vi "Server_API_Call.vi"(6 "Server":path, 7 "Direction":enum16{"ASK", "TELL"}(ring), 8 "error in (no error)":errorcluster, 9 "Payload":string, 11 "cmd":string) -> (0 "error out":errorcluster, 1 "Running?":bool, 2 "Send to Server":string, 3 "Read from Server":string)   [LabVIEW 2020]
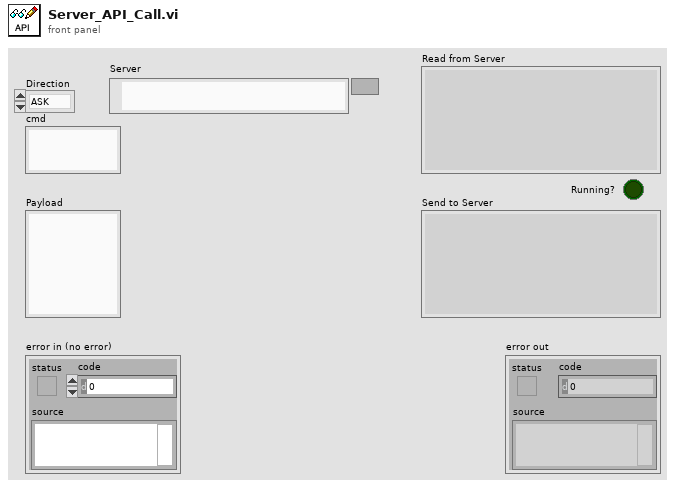
[diagram p1: front panel]
types:
  T1 = enum32{"Bad", "Idle", "Run top level", "Running"}
  T2 = enum32{"Invalid", "Standard", "Closed", "Hidden", "Minimized", "Maximized"}
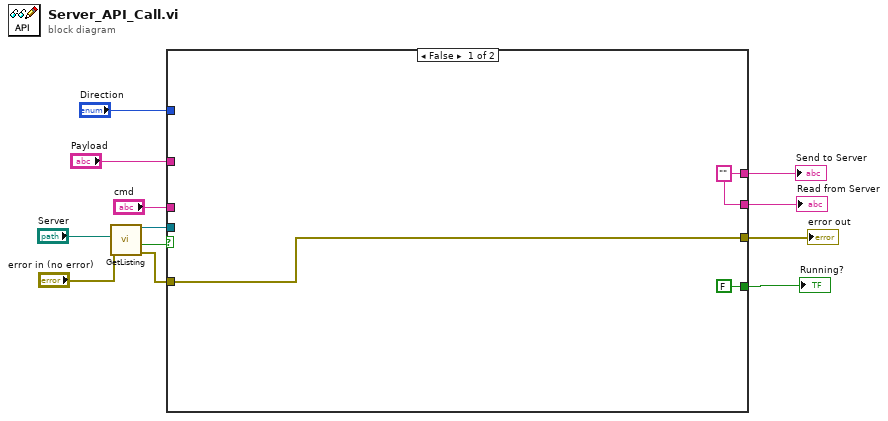
[diagram p0: block diagram]
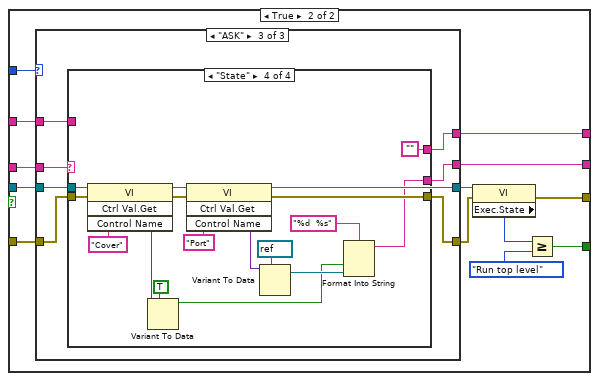
[diagram p2: hidden frame]
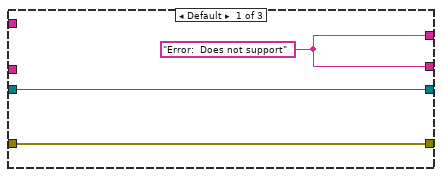
[diagram p3: hidden frame]
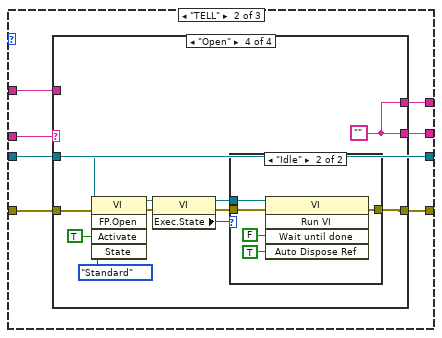
[diagram p4: hidden frame]
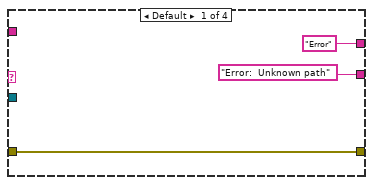
[diagram p5: hidden frame]
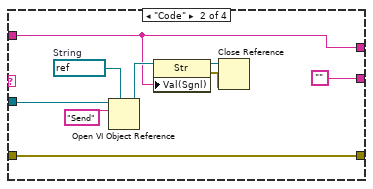
[diagram p6: hidden frame]
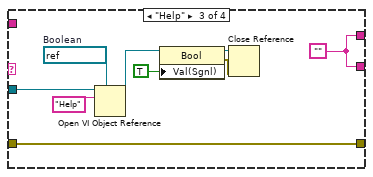
[diagram p7: hidden frame]
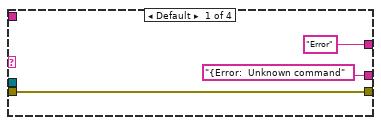
[diagram p9: hidden frame]
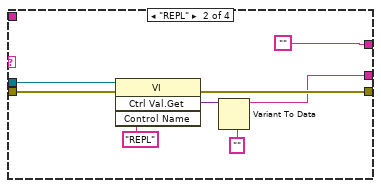
[diagram p10: hidden frame]
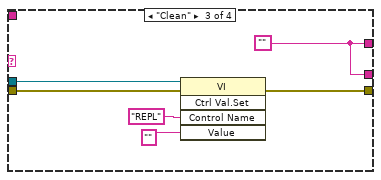
[diagram p11: hidden frame]
diagram:
  n1 = call "GetListing.vi"("error in (no error)"="error in (no error)", "Server"="Server") -> ("error out"=w4:errorcluster, "Found"=w1:bool, "VI out"=w9:refnum<vi>)  [unwired: 7 in]
  n2 = case shown="False" w1 {
    tunnel: [w15 w28] -> w12
    tunnel: [w15 w27] -> w11
    tunnel: w9 -> [_ w26]
    tunnel: "Direction" -> [_ w25]
    tunnel: "Payload" -> [_ w24]
    tunnel: "cmd" -> [_ w23]
    tunnel: w4 -> [w14 w22]
    tunnel: [FALSE w17] -> w3
    tunnel: [w14 w16] -> w2
    frame False {
      w15 = "" ("input 2")
    }
    frame True {
      n3 = case shown="\"ASK\"" w25 {
        tunnel: [w31 w38 w83] -> w28
        tunnel: w24 -> [_ w37 w82]
        tunnel: [w31 w36 w81] -> w27
        tunnel: w26 -> [w29 w32 w77]
        tunnel: w22 -> [w30 w35 w80]
        tunnel: [w30 w34 w79] -> w20
        tunnel: w23 -> [_ w33 w78]
        tunnel: [w29 w32 w77] -> w21
        frame Default {
          w31 = "Error:  Does not support" ("input 2")
        }
        frame "TELL" {
          n4 = case shown="\"Open\"" w33 {
            tunnel: ["Error:  Unknown path" ("input 2") "" w51 w68] -> w38
            tunnel: w37 -> [_ w44 _ _]
            tunnel: ["Error" ("input 2") w44 w51 w68] -> w36
            tunnel: w35 -> [w39 w49 w59 w66]
            tunnel: [w39 w49 w59 w60] -> w34
            tunnel: w32 -> [_ w46 w56 w67]
            frame Default {
            }
            frame "Code" {
              w48 = refnum<vi> refnum  # String
              n5 = Open VI Object Reference(7:w48, 10:"Send" ("name/order"), 11:w46) -> (3:w45:refnum<vi>)  [unwired: 1 in, 1 out]
              n6 = property class="Str"(reference=w45, "Val(Sgnl)"=w44) -> (reference out=w42:refnum<vi>, error out=w43:errorcluster)  [unwired: 1 in]
              n7 = Close Reference(reference=w42, error in (no error)=w43) -> ()  [unwired: 1 out]
            }
            frame "Help" {
              w58 = refnum<vi> refnum  # Boolean
              w51 = ""
              n8 = Open VI Object Reference(7:w58, 10:"Help" ("name/order"), 11:w56) -> (3:w55:refnum<vi>)  [unwired: 1 in, 1 out]
              n9 = property class="Bool"(reference=w55, "Val(Sgnl)"=TRUE) -> (reference out=w53:refnum<vi>, error out=w54:errorcluster)  [unwired: 1 in]
              n10 = Close Reference(reference=w53, error in (no error)=w54) -> ()  [unwired: 1 out]
            }
            frame "Open" {
              w68 = ""
              n11 = invoke class="VI" method="FP.Open"(reference=w67, error in=w66, "Activate"=TRUE ("Activate?"), "State"=T2."Standard" ("Front Panel Window:State")) -> (reference out=w65:refnum<vi>, error out=w64:errorcluster)  [unwired: 1 in, 3 out]
              n12 = property class="VI"(reference=w65, error in=w64) -> (reference out=w62:refnum<vi>, error out=w61:errorcluster, "Exec.State"=w63:T1)
              n13 = case shown="\"Idle\"" w63 {
                tunnel: w62 -> [_ w76]
                tunnel: w61 -> [w71 w75]
                tunnel: [w71 w74] -> w60
                frame Default {
                }
                frame "Idle" {
                  n14 = invoke class="VI" method="Run VI"(reference=w76, error in=w75, "Wait until done"=FALSE ("Activate?"), "Auto Dispose Ref"=TRUE ("Activate?")) -> (error out=w74:errorcluster)  [unwired: 1 in, 4 out]
                }
              }
            }
          }
        }
        frame "ASK" {
          n15 = case shown="\"State\"" w78 {
            tunnel: ["{Error:  Unknown command" ("input 2") w87 w100 w101] -> w83
            tunnel: w82 -> [_ _ _ _]
            tunnel: ["Error" ("input 2") "" w100 ""] -> w81
            tunnel: w77 -> [_ w89 w97 w109]
            tunnel: w80 -> [w84 w90 w96 w108]
            tunnel: [w84 w88 w95 w105] -> w79
            frame Default {
            }
            frame "REPL" {
              n16 = invoke class="VI" method="Ctrl Val.Get"(reference=w89, error in=w90, "Control Name"="REPL") -> (error out=w88:errorcluster, "Get Control Value Variant"=w92:variant)  [unwired: 1 in, 2 out]
              n17 = Variant To Data(type="" ("Control Name"), Variant=w92) -> (data=w87:string)  [unwired: 1 in, 1 out]
            }
            frame "Clean" {
              w100 = ""
              n18 = invoke class="VI" method="Ctrl Val.Set"(reference=w97, error in=w96, "Control Name"="REPL", "Value"="" ("Control Name")) -> (error out=w95:errorcluster)  [unwired: 1 in, 4 out]
            }
            frame "State" {
              n19 = invoke class="VI" method="Ctrl Val.Get"(reference=w109, error in=w108, "Control Name"="Cover") -> (reference out=w107:refnum<vi>, error out=w106:errorcluster, "Get Control Value Variant"=w110:variant)  [unwired: 1 in, 1 out]
              n20 = Variant To Data(type=TRUE, Variant=w110) -> (data=w102:bool)  [unwired: 1 in, 1 out]
              n21 = invoke class="VI" method="Ctrl Val.Get"(reference=w107, error in=w106, "Control Name"="Port") -> (error out=w105:errorcluster, "Get Control Value Variant"=w111:variant)  [unwired: 1 in, 2 out]
              n22 = Variant To Data(type=refnum<visa-resource-name> refnum ("Port"), Variant=w111) -> (data=w104:refnum<visa-resource-name>)  [unwired: 1 in, 1 out]
              n23 = Format Into String(format string="%d  %s", w102, w104) -> (resulting string=w101:string)  [unwired: 2 in, 1 out]
            }
          }
        }
      }
      n24 = property class="VI"(reference=w21, error in=w20) -> (error out=w16:errorcluster, "Exec.State"=w19:T1)  [unwired: 1 out]
      n25 = Greater Or Equal?(x=w19, y=T1."Run top level" ("Execution:State")) -> (x >= y?=w17:bool)
    }
  }
  "error out" <- w2
  "Read from Server" <- w12
  "Send to Server" <- w11
  "Running?" <- w3
